vi "Calculator Brainstorming V2.vi"() -> ()   [LabVIEW 2017]
panel:
  in  "=":bool
  in  ".":bool
  in  "÷":bool
  in  "x":bool
  in  "-":bool
  in  "+":bool
  in  "9":bool
  in  "8":bool
  in  "7":bool
  in  "0":bool
  in  "6":bool
  in  "CLEAR":bool
  in  "?":bool
  in  "1":bool
  in  "5":bool
  in  "4":bool
  in  "3":bool
  in  "2":bool
  out "Display":dbl
  # "Don't work:"
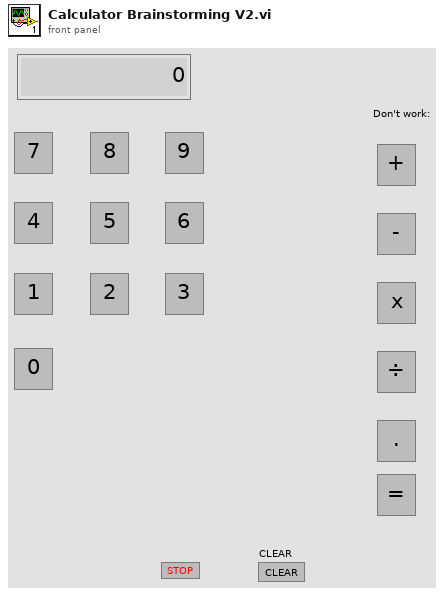
[diagram p1: front panel]
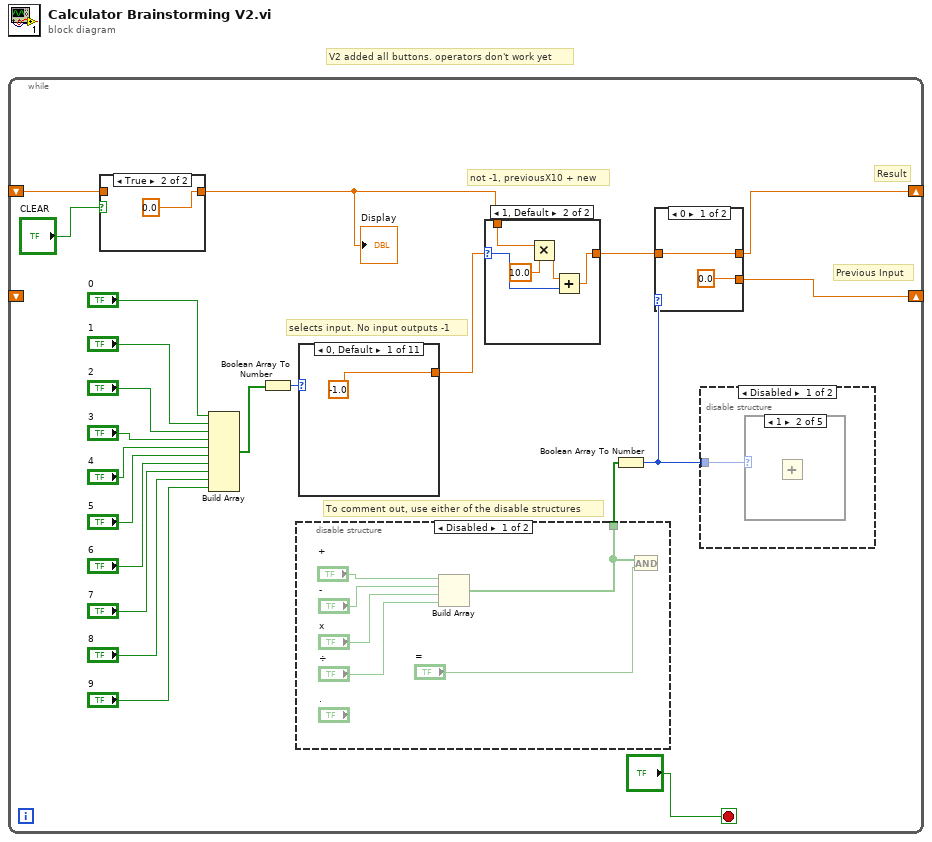
[diagram p0: block diagram]
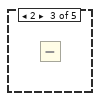
[diagram p3: hidden frame]
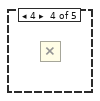
[diagram p4: hidden frame]
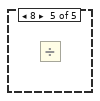
[diagram p5: hidden frame]
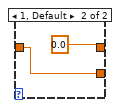
[diagram p8: hidden frame]
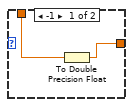
[diagram p10: hidden frame]
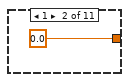
[diagram p11: hidden frame]
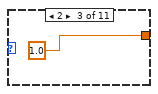
[diagram p12: hidden frame]
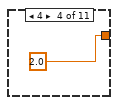
[diagram p13: hidden frame]
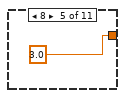
[diagram p14: hidden frame]
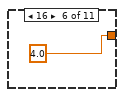
[diagram p15: hidden frame]
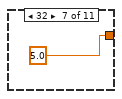
[diagram p16: hidden frame]
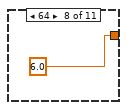
[diagram p17: hidden frame]
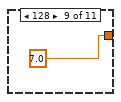
[diagram p18: hidden frame]
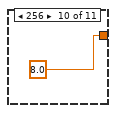
[diagram p19: hidden frame]
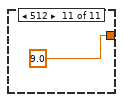
[diagram p20: hidden frame]
diagram:
  # "V2 added all buttons. operators don't work yet"
  n1 = while {
    shift-right: [w4] -> _
    shift-left: _ -> [w18]
    shift-right: [w3] -> _
    shift-left: _ -> [_]
    stop <- "?" stop-if-true
    # "To comment out, use either of the disable structures"
    # "not -1, previousX10 + new"
    # "selects input. No input outputs -1"
    # "Previous Input"
    # "Result"
    n2 = case shown="True" "CLEAR" {
      tunnel: [w34 0.0] -> w19
      tunnel: w18 -> [w34 _]
      frame False {
      }
      frame True {
      }
    }
    "Display" <- w19
    n3 = Build Array("0", "1", "2", "3", "4", "5", "6", "7", "8", "9") -> (w16:bool[])
    n4 = Boolean Array To Number(Boolean array=w16) -> (number=w22:u32)
    n5 = disable-structure shown="Disabled" {
      disable-tunnel: [w24 _] -> w2
      frame Disabled {
        n6 = Build Array("+", "-", "x", "÷") -> (w24:bool[])
        n7 = And(x=w24, y="=") -> ()  [unwired: 1 out]
      }
      frame Enabled {
      }
    }
    n8 = case shown="0, Default" w22 {
      tunnel: [-1.0 0.0 1.0 2.0 3.0 4.0 5.0 6.0 7.0 8.0 9.0] -> w21
      frame 0, Default {
      }
      frame 1 {
      }
      frame 2 {
      }
      frame 4 {
      }
      frame 8 {
      }
      frame 16 {
      }
      frame 32 {
      }
      frame 64 {
      }
      frame 128 {
      }
      frame 256 {
      }
      frame 512 {
      }
    }
    n9 = case shown="1, Default" w21 {
      selector: w21 -> [_ w41]
      tunnel: [w36 w38] -> w5
      tunnel: w19 -> [w37 w39]
      frame -1 {
        n10 = To Double Precision Float(number=w37) -> (double precision float=w36:dbl)
      }
      frame 1, Default {
        n11 = Multiply(x=w39, y=10.0) -> (x*y=w42:dbl)
        n12 = Add(x=w42, y=w41) -> (x+y=w38:dbl)
      }
    }
    n13 = Boolean Array To Number(Boolean array=w2) -> (number=w1:u32)
    n14 = case shown="0" w1 {
      tunnel: [w31 0.0] -> w4
      tunnel: w5 -> [w31 w33]
      tunnel: [0.0 w33] -> w3
      frame 0 {
      }
      frame 1, Default {
      }
    }
    n15 = disable-structure shown="Disabled" {
      disable-tunnel: w1 -> [w23 _]
      frame Disabled {
        n16 = case shown="1" w23 {
          frame 0, Default {
          }
          frame 1 {
            n17 = Add() -> ()  [unwired: 2 in, 1 out]
          }
          frame 2 {
            n18 = Subtract() -> ()  [unwired: 2 in, 1 out]
          }
          frame 4 {
            n19 = Multiply() -> ()  [unwired: 2 in, 1 out]
          }
          frame 8 {
            n20 = Divide() -> ()  [unwired: 2 in, 1 out]
          }
        }
      }
      frame Enabled {
      }
    }
  }
